vi "timeout.vi"(8 "error in (no error)":errorcluster, 9 "timeout_secs":u64, 10 "connect_timeout_secs":u64, 11 "ClientBuilder in":refnum<class "ClientBuilder.lvclass">) -> (0 "error out":errorcluster, 2 "success":bool, 3 "ClientBuilder out":refnum<class "ClientBuilder.lvclass">)   [LabVIEW 2020, in "reqwest.lvlib" / "ClientBuilder.lvclass"]
uses:
  ClientBuilder.lvclass
  ClientBuilder.lvclass/ClientBuilder.ctl
  lv_reqwest_64.so
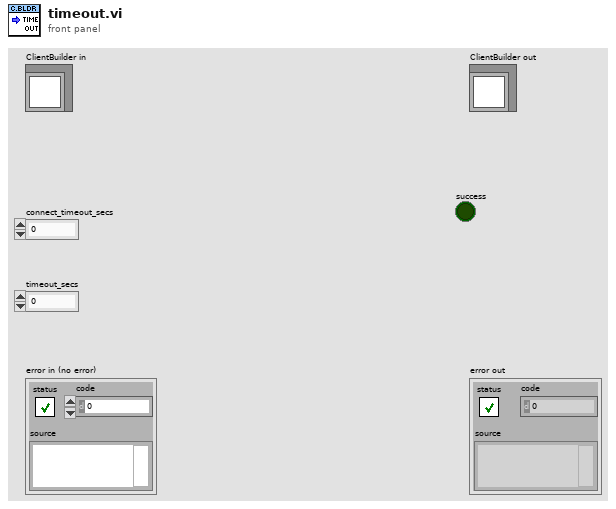
[diagram p1: front panel]
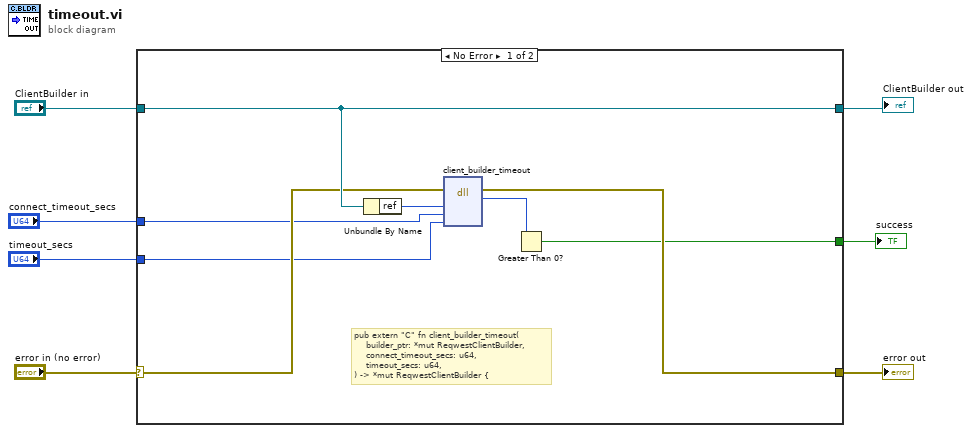
[diagram p0: block diagram]
diagram:
  n1 = case shown="No Error" "error in (no error)" {
    selector: "error in (no error)" -> [w12 w16]
    tunnel: "ClientBuilder in" -> [w13 w17]
    tunnel: [w15 w16] -> w4
    tunnel: [w13 w17] -> w5
    tunnel: "connect_timeout_secs" -> [w11 _]
    tunnel: "timeout_secs" -> [w10 _]
    tunnel: [w8 _] -> w1
    frame No Error {
      # "pub extern \"C\" fn client_builder_timeout(\n    builder_ptr: *mut ReqwestClientBuilder,\n    connect_timeout_secs: u64,\n    timeout_secs: u64,\n) -> *mut ReqwestClientBuilder {"
      n2 = Unbundle By Name(w13) -> ("ref"=w14:u64)
      n3 = dll-call lib="home/jim-kring/Projects/reqwest-rs-labview/lv_src/lv_reqwest_*.*" fn="client_builder_timeout"(error in=w12, "client_builder_ref"=w14, "connect_timeout_secs"=w11, "timeout_secs"=w10) -> (error out=w15:errorcluster, "success"=w9:u8)  [unwired: 5 in, 1 out]
      n4 = Greater Than 0?(x=w9) -> (x > 0?=w8:bool)
    }
    frame Error {
    }
  }
  "error out" <- w4
  "ClientBuilder out" <- w5
  "success" <- w1
